vi "USRP Rx Init.vi"(2 "setup para":T1={"Active Antenna"="RX2", "Carrier Frequency"=0.0, "IQ Rate"=0.0, "Gain"=0.0}, 3 "device names":refnum<k15>="192.168.10.2") -> (0 "error out":errorcluster, 1 "session handle out":refnum<k15>)   [LabVIEW 2014]
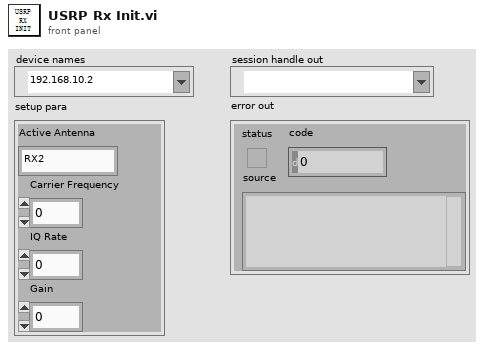
[diagram p1: front panel]
types:
  T1 = cluster{"Active Antenna":string, "Carrier Frequency":dbl, "IQ Rate":dbl, "Gain":dbl}
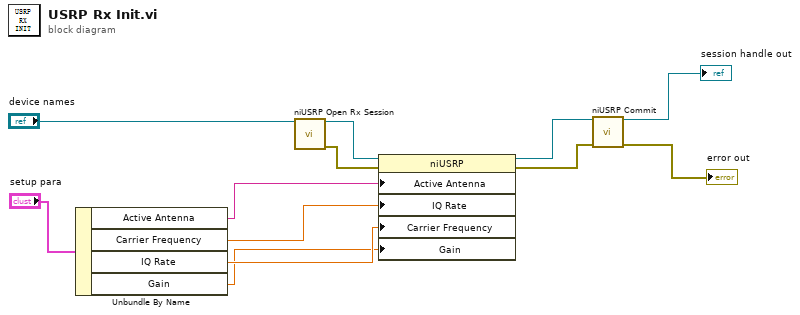
[diagram p0: block diagram]
diagram:
  n1 = Unbundle By Name("setup para") -> ("Active Antenna"=w8:string, "Carrier Frequency"=w7:dbl, "IQ Rate"=w6:dbl, "Gain"=w5:dbl)
  n2 = call <instrlib>:"niUSRP Open Rx Session.vi"("device names"="device names") -> ("session handle out"=w11:refnum<k15>, "error out"=w10:errorcluster)  [unwired: 13 in]
  n3 = property class="niUSRP"(reference=w11, error in=w10, "Active Antenna"=w8, "IQ Rate"=w7, "Carrier Frequency"=w6, "Gain"=w5) -> (reference out=w4:refnum<k15>, error out=w3:errorcluster)
  n4 = call <instrlib>:"niUSRP Commit.vi"("session handle"=w4, "error in (no error)"=w3) -> ("session handle out"=→"session handle out":refnum<k15>, "error out"=→"error out":errorcluster)  [unwired: 12 in]
